vi "ExposureStatusMessage.vi"(0 "ExposureFlag":string) -> (1 "Message":string, 2 "Exposing":bool)   [LabVIEW 2014]
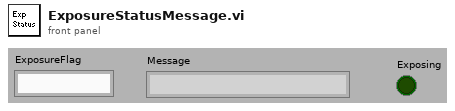
[diagram p1: front panel]
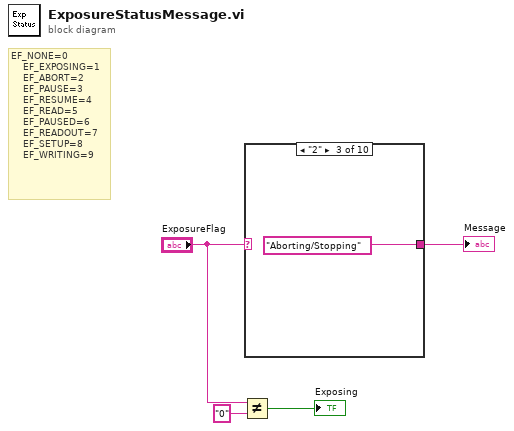
[diagram p0: block diagram]
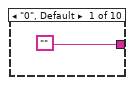
[diagram p2: hidden frame]
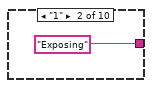
[diagram p3: hidden frame]
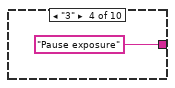
[diagram p4: hidden frame]
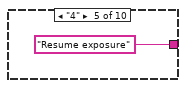
[diagram p5: hidden frame]
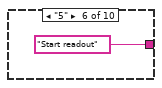
[diagram p6: hidden frame]
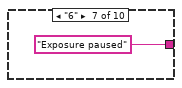
[diagram p7: hidden frame]
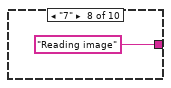
[diagram p8: hidden frame]
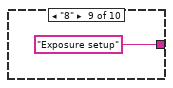
[diagram p9: hidden frame]
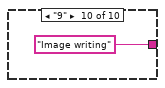
[diagram p10: hidden frame]
diagram:
  # "EF_NONE=0\n    EF_EXPOSING=1\n    EF_ABORT=2\n    EF_PAUSE=3\n    EF_RESUME=4\n    EF_READ=5\n    EF_PAUSED=6\n    EF_READOUT=7\n    EF_SETUP=8\n    EF_WRITING=9"
  n1 = Not Equal?(x="ExposureFlag", y="0") -> (x != y?=→"Exposing":bool)
  n2 = case shown="\"2\"" "ExposureFlag" {
    tunnel: ["" "Exposing" ("Message") "Aborting/Stopping" ("Message") "Pause exposure" ("Message") "Resume exposure" ("Message") "Start readout" ("Message") "Exposure paused" ("Message") "Reading image" ("Message") "Exposure setup" ("Message") "Image writing" ("Message")] -> w4
    frame "0", Default {
    }
    frame "1" {
    }
    frame "2" {
    }
    frame "3" {
    }
    frame "4" {
    }
    frame "5" {
    }
    frame "6" {
    }
    frame "7" {
    }
    frame "8" {
    }
    frame "9" {
    }
  }
  "Message" <- w4
